vi "ChannelUI.vi"() -> ()   [LabVIEW 2014, in "Channel.lvclass"]
doc: "Template for creating new user-interface VIs for inherited classes."
uses:
  Channel.lvclass
  <vilib>/NI/AMC/Message Queue.ctl
  <vilib>/NI/AMC/Message.ctl
  <vilib>/NI/Tools/Keyed Array/KeyedArray.ctl
  xCE/xceTreeObj/xceTreeObj.lvclass
  channel_dataType.ctl
  _Shared/Symbols/enum_Symbols.ctl
  Channel.lvclass/Channel.ctl
  Channel_FXP/Channel_FXP.lvclass
  Channel_FXP/Channel_FXP.lvclass/Channel_FXP.ctl
  xCE/_shared/replaceNode.ctl
  xCE/xceDataNode/xceDataNode.lvclass
  <vilib>/NI/AMC/Read Termination Message.vi
  <vilib>/NI/AMC/Create Single Message.vi
  <vilib>/NI/AMC/Update Message Routing Info.vi
  <vilib>/NI/AMC/Globals.vi
  <vilib>/NI/AMC/Send Message.vi
  <vilib>/NI/AMC/AMC.lvlib
  xCE/xceNode/xceNode.lvclass
  <vilib>/NI/Tools/Keyed Array/Tools_KeyedArray.lvlib
panel:
  in  "View Mode":enum32{"Channel", "Parameter"}(tab)
  in  "Offset":dbl format="%#_12g"
  in  "Scale":dbl format="%#_12g"
  in  "Set Scale and Offset":bool
  in  "Description":string
  in  "Category":string="Default"
  in  "Name":string
  in  "Symbol":T1
  in  "Unit":string
  in  "Channel Specific":enum32{"Basic", "FXP"}(tab)
  in  "FXP Integer Length":i32
  in  "FXP - Word Length":i32
  in  "Parameter":T2
  in  "Data Type":T3
  in  "DataNode*":refnum<data-value>
  in  "AMC*":T4
  in  "Exit":bool
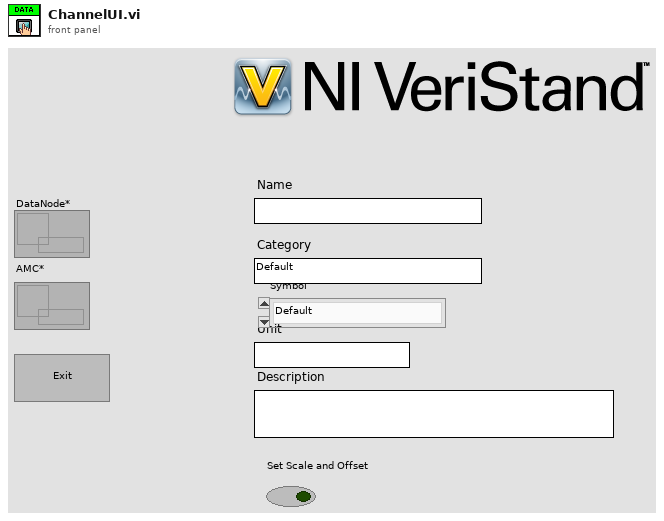
[diagram p1: front panel]
types:
  T1 = typedef "enum_Symbols.ctl" = enum16{"Default", "Analog Input", "Analog Output", "Digital Input", "Digital Output", "PWM Input", "PWM Output"}
  T2 = cluster{"Name":string, "Control Name":string, "Initial Value":dbl, "Scale":dbl, "Offset":dbl}
  T3 = typedef "Channel.lvclass/channel_dataType.ctl" = enum16{"Boolean", "U8", "I8", "U16", "I16", "U32", "I32", "U64", "I64", "FXPI32", "FXPU32", "FXPI64", "FXPU64", "PWM"}
  T4 = typedef "AMC.lvlib/Message Queue.ctl" = refnum<queue>
  T5 = typedef "replaceNode.ctl" = cluster{"ToReplaceNode*":refnum<data-value>, "Replace Class":string}
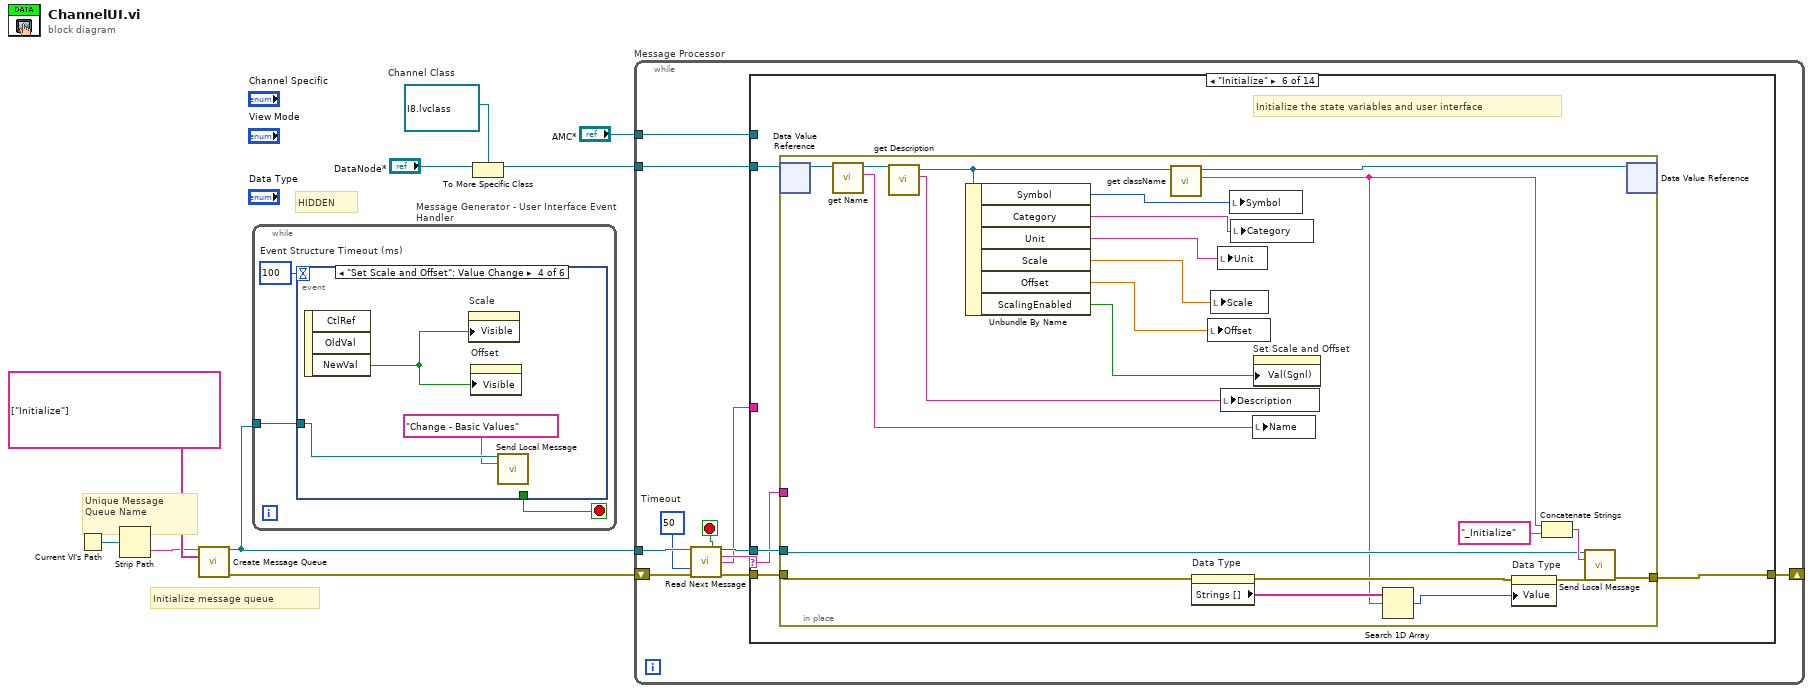
[diagram p0: block diagram]
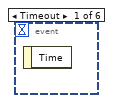
[diagram p2: hidden frame]
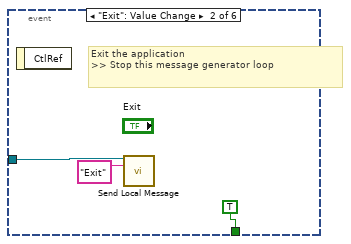
[diagram p3: hidden frame]
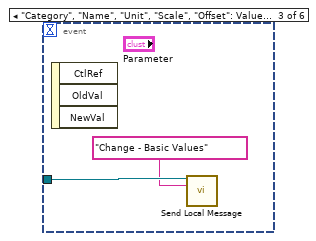
[diagram p4: hidden frame]
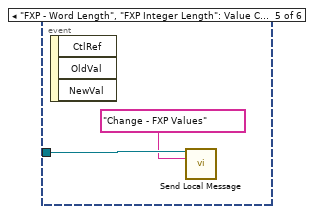
[diagram p5: hidden frame]
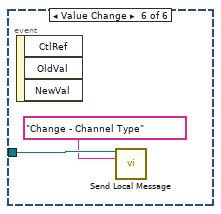
[diagram p6: hidden frame]
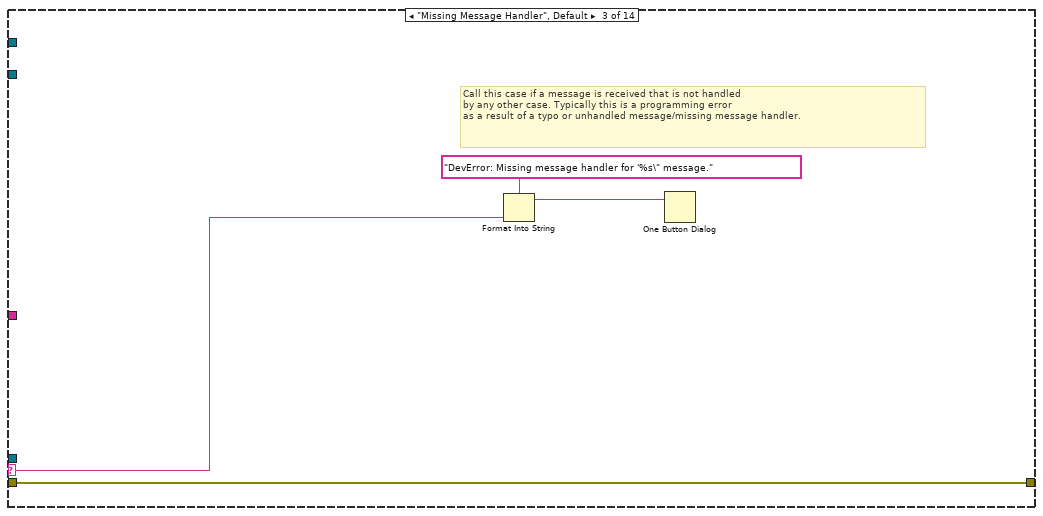
[diagram p9: hidden frame]
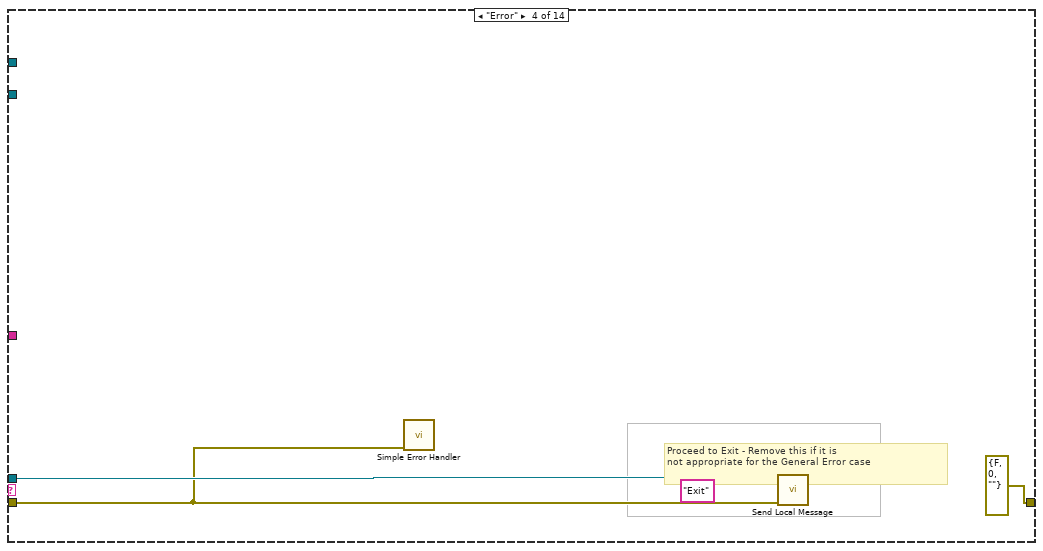
[diagram p10: hidden frame]
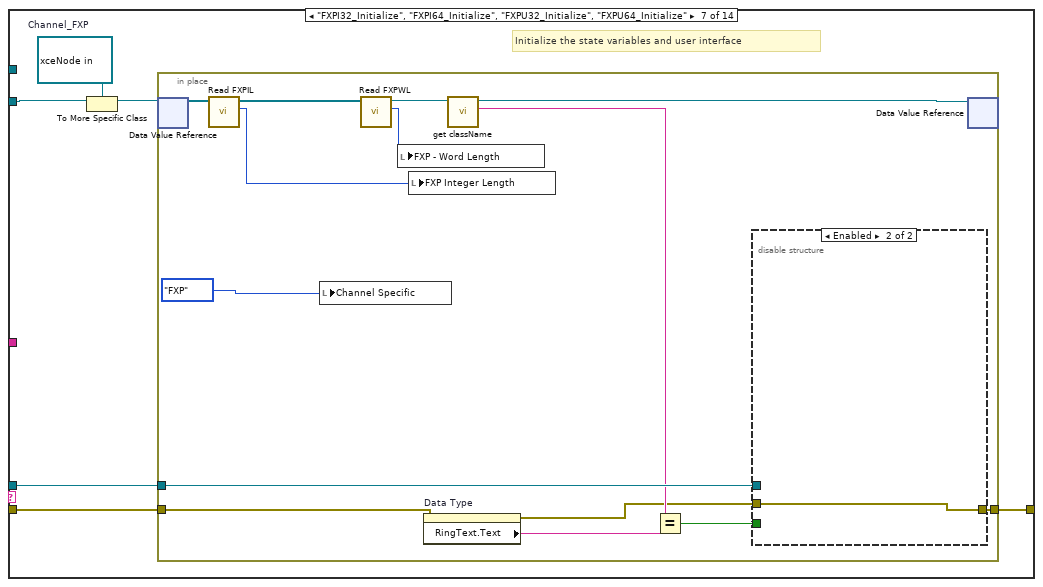
[diagram p12: hidden frame]
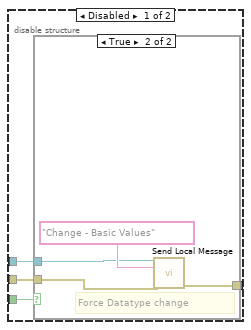
[diagram p13: hidden frame]
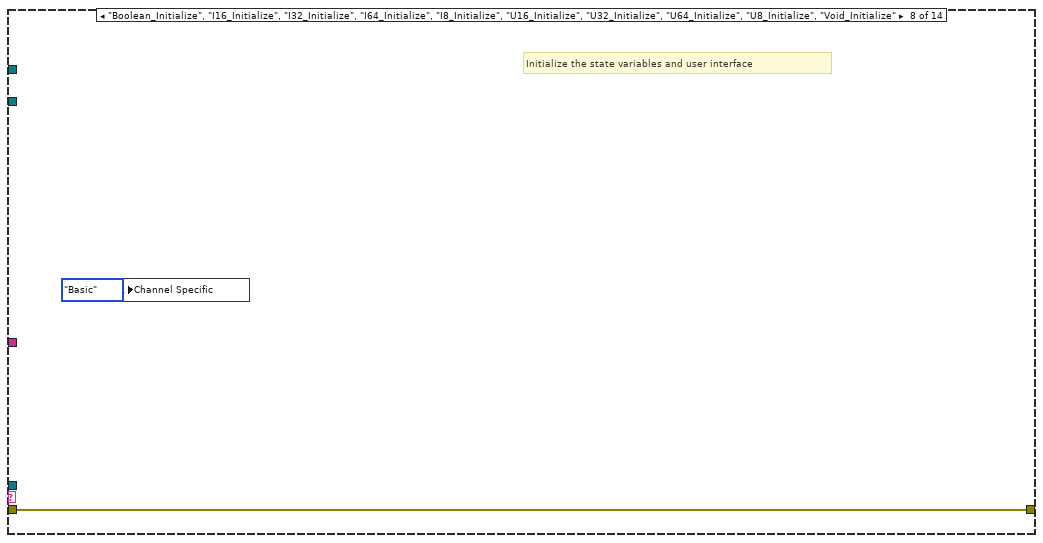
[diagram p15: hidden frame]
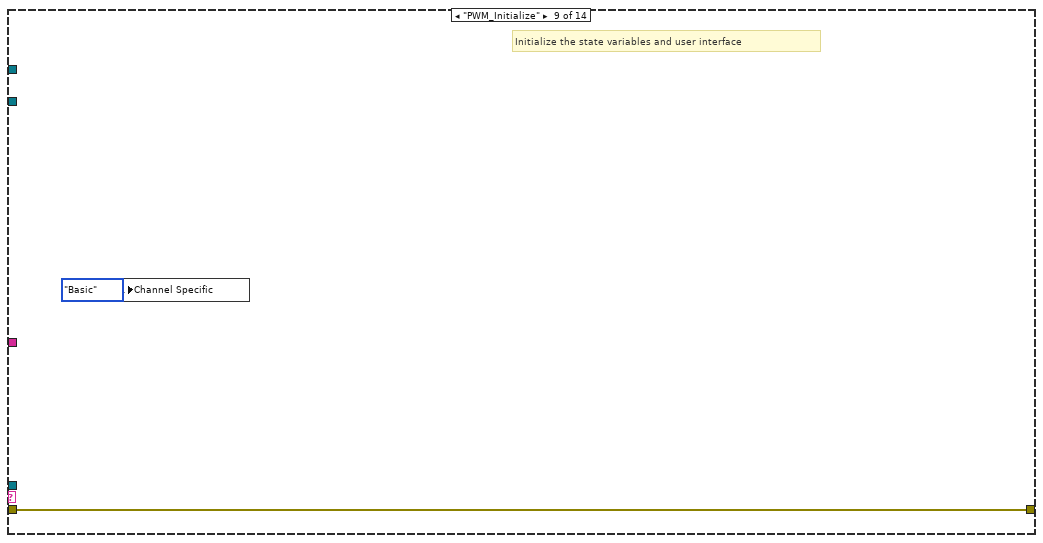
[diagram p16: hidden frame]
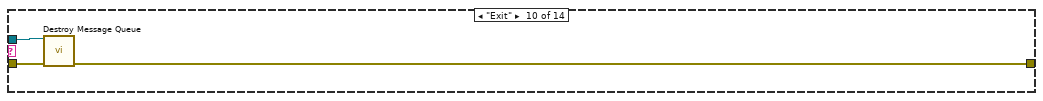
[diagram p17: hidden frame]
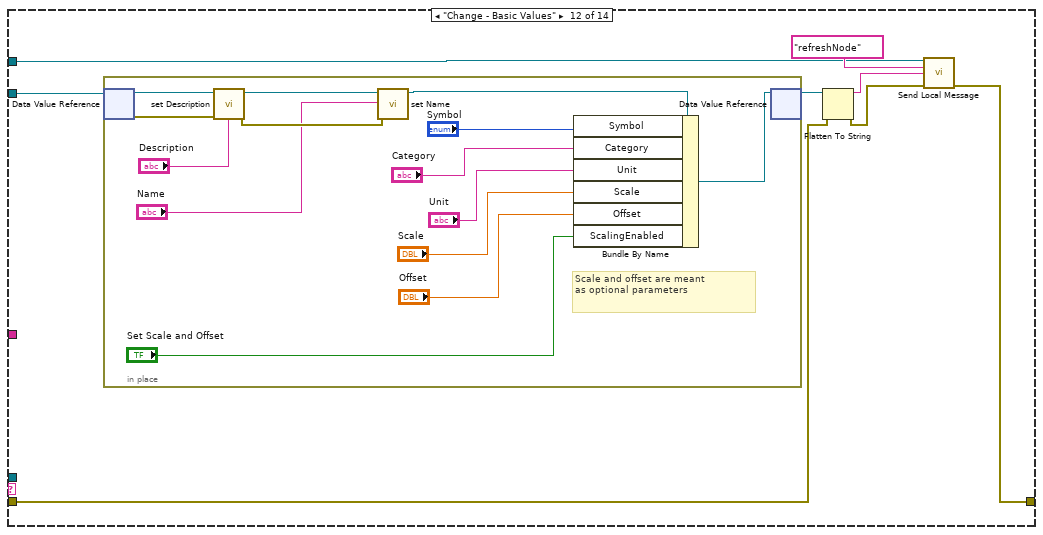
[diagram p19: hidden frame]
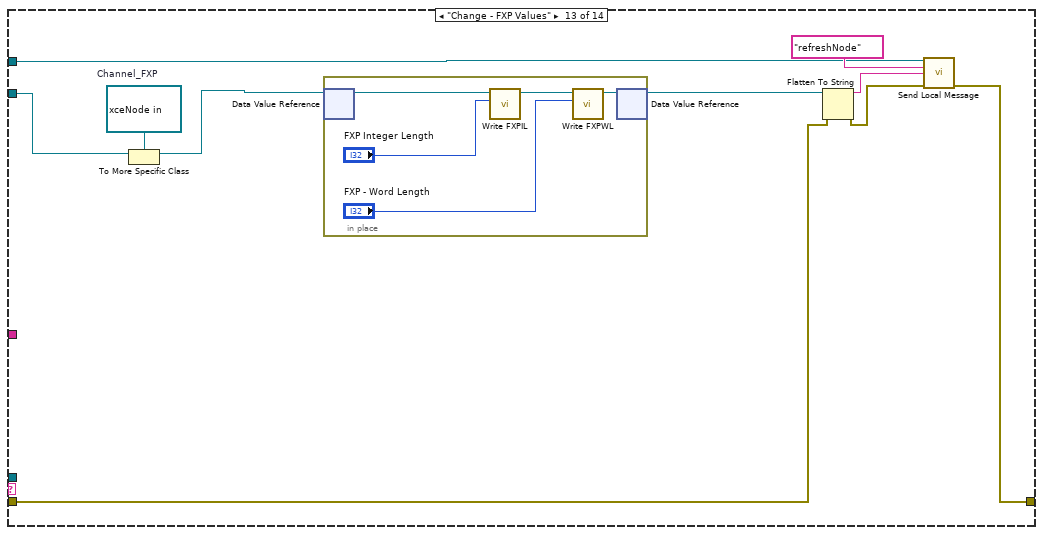
[diagram p20: hidden frame]
diagram:
  w1 = refnum<data-value> refnum  # Channel Class
  # "HIDDEN"
  # "Initialize message queue"
  # "Unique Message\nQueue Name"
  n1 = Current VI's Path() -> (path=w5:path)
  n2 = Strip Path(path=w5) -> (name=w8:string)  [unwired: 1 out]
  n3 = call <vilib>:"Create Message Queue.vi"("message queue name"=w8, "initial message names"=string[] ["Initialize"]) -> ("message queue out"=w7:T4, "error out"=w6:errorcluster)  [unwired: 12 in]
  n4 = while "Message Generator - User Interface Event Handler" {
    tunnel: w7 -> [w10]
    stop <- w11 stop-if-true
    w12 = 100  # Event Structure Timeout (ms)
    n5 = event shown="[3] \"Set Scale and Offset\": Value Change" {
      selector: _ -> [_ _ _ _ _ _]
      dyn-events: _ -> [_ _ _ _ _ _]
      timeout: w12 -> [_ _ _ _ _ _]
      tunnel: [_ TRUE ("Discard?") _ _ _ _] -> w11
      tunnel: w10 -> [_ w13 w17 w19 w22 w24]
      event Timeout {
        n6 = event-data() -> ()  [unwired: 2 out]
      }
      event "Exit": Value Change {
        # "Exit the application\n>> Stop this message generator loop"
        n7 = event-data() -> ()  [unwired: 2 out]
        n8 = call <vilib>:"Send Local Message.vi"("message queue in"=w13, "message name"="Exit") -> ()  [unwired: 11 in, 3 out]
      }
      event "Category", "Name", "Unit", "Scale", "Offset": Value Change {
        n9 = event-data() -> ()  [unwired: 4 out]
        n10 = call <vilib>:"Send Local Message.vi"("message queue in"=w17, "message name"="Change - Basic Values" ("Message Name")) -> ()  [unwired: 11 in, 3 out]
      }
      event "Set Scale and Offset": Value Change {
        n11 = event-data() -> ("NewVal"=w20:bool)  [unwired: 3 out]
        n12 = property on="Scale" class="DigNum (strict)"("Visible"=w20) -> ()  [unwired: 2 in, 2 out]
        n13 = property on="Offset" class="DigNum (strict)"("Visible"=w20) -> ()  [unwired: 2 in, 2 out]
        n14 = call <vilib>:"Send Local Message.vi"("message queue in"=w19, "message name"="Change - Basic Values" ("Message Name")) -> ()  [unwired: 11 in, 3 out]
      }
      event "FXP - Word Length", "FXP Integer Length": Value Change {
        n15 = event-data() -> ()  [unwired: 4 out]
        n16 = call <vilib>:"Send Local Message.vi"("message queue in"=w22, "message name"="Change - FXP Values" ("Message Name")) -> ()  [unwired: 11 in, 3 out]
      }
      event Value Change {
        n17 = event-data() -> ()  [unwired: 4 out]
        n18 = call <vilib>:"Send Local Message.vi"("message queue in"=w24, "message name"="Change - Channel Type" ("Message Name")) -> ()  [unwired: 11 in, 3 out]
      }
    }
  }
  n19 = To More Specific Class(target class=w1, reference="DataNode*") -> (specific class reference=w2:refnum<data-value>)  [unwired: 1 in, 1 out]
  n20 = while "Message Processor" {
    shift-left: w6 -> [w32]
    shift-right: [w25] -> _
    tunnel: w7 -> [w33]
    tunnel: "AMC*" -> [w26]
    tunnel: w2 -> [w27]
    stop <- w35 stop-if-true
    w30 = 50  # Timeout
    n21 = call <vilib>:"Read Next Message.vi"("message queue in"=w33, "timeout (1 ms)"=w30, "error in"=w32) -> ("exit process?"=w35:bool, "message queue out"=w34:T4, "message name"=w29:string, "message value"=w28:string, "error out"=w31:errorcluster)  [unwired: 5 in, 3 out]
    n22 = case shown="\"Initialize\"" w29 {
      selector: w29 -> [_ _ w41 _ _ w47 _ _ _ _ _ _ _ _]
      tunnel: w34 -> [_ _ _ w45 _ w49 w78 _ _ w109 _ _ _ _]
      tunnel: w31 -> [w36 w37 w38 w43 w46 w50 w79 w105 w107 w110 w111 w113 w138 w151]
      tunnel: w28 -> [_ _ _ _ _ _ _ _ _ _ _ _ _ _]
      tunnel: w27 -> [_ _ _ _ _ w51 w77 _ _ _ _ w119 w135 w157]
      tunnel: w26 -> [_ _ _ _ _ _ _ _ _ _ _ w115 w140 w155]
      tunnel: [w36 w37 w38 errorcluster {"status"=FALSE, "code"=0, "source"=""} ("error out") w46 w48 w74 w105 w107 w108 w111 w112 w137 w152] -> w25
      frame "---------- Framework Operations ----------" {
        # "Dummy case to add a seperator in the Case Structure menu"
      }
      frame "", "Idle" {
      }
      frame "Missing Message Handler", Default {
        # "Call this case if a message is received that is not handled \nby any other case. Typically this is a programming error\nas a result of a typo or unhandled message/missing message handler."
        n23 = Format Into String(format string="DevError: Missing message handler for '%s\" message." ("message"), w41) -> (resulting string=w39:string)  [unwired: 2 in, 1 out]
        n24 = One Button Dialog(message=w39) -> ()  [unwired: 2 out]
      }
      frame "Error" {
        # "Proceed to Exit - Remove this if it is\nnot appropriate for the General Error case"
        n25 = call <vilib>:"Simple Error Handler.vi"("error in (no error)"=w43) -> ()  [unwired: 1 in, 8 out]
        n26 = call <vilib>:"Send Local Message.vi"("message queue in"=w45, "message name"="Exit", "error in"=w43) -> ()  [unwired: 10 in, 3 out]
      }
      frame "---------- Generic Operations ----------" {
        # "Dummy case to add a seperator in the Case Structure menu"
      }
      frame "Initialize" {
        # "Initialize the state variables and user interface"
        n27 = in-place {
          in-place-border: w50 -> [w60]
          in-place-border: w49 -> [w62]
          in-place-border: [w61] -> w48
          in-place-border: w47 -> [_]
          n28 = in-place-dvr #1(w51) -> (w68:refnum<class "Channel.lvclass">)  [unwired: 1 out]
          n29 = call "get Name.vi"("xceDataNode in"=w68) -> ("Name"=w72:string, "xceDataNode out"=w73:refnum<class "Channel.lvclass">)  [unwired: 8 in, 1 out]
          n30 = call "get Description.vi"("xceDataNode in"=w73) -> ("Description"=w71:string, "xceDataNode out"=w67:refnum<class "Channel.lvclass">)  [unwired: 8 in, 1 out]
          n31 = Unbundle By Name(w67) -> ("Symbol"=w70:T1, "Category"=w69:string, "Unit"=w65:string, "Scale"=w53:dbl, "Offset"=w54:dbl, "ScalingEnabled"=w52:bool)
          n32 = call "get className.vi"("xceNode in"=w67) -> ("Class name"=w55:string, "xceNode out"=w66:refnum<class "Channel.lvclass">)  [unwired: 8 in, 1 out]
          n33 = property on="Data Type" class="Enum (strict)"(error in=w60) -> (error out=w58:errorcluster, "Strings []"=w59:string[])  [unwired: 1 in, 1 out]
          n34 = local write "Offset"(w54) -> ()
          n35 = local write "Scale"(w53) -> ()
          n36 = local write "Unit"(w65) -> ()
          n37 = local write "Description"(w71) -> ()
          n38 = local write "Symbol"(w70) -> ()
          n39 = local write "Category"(w69) -> ()
          n40 = local write "Name"(w72) -> ()
          n41 = property on="Set Scale and Offset" class="Bool (strict)"("Val(Sgnl)"=w52) -> ()  [unwired: 2 in, 2 out]
          n42 = Search 1D Array(1D array=w59, element=w55) -> (index of element=w57:i32)  [unwired: 1 in]
          n43 = property on="Data Type" class="Enum (strict)"(error in=w58, "Value"=w57) -> (error out=w56:errorcluster)  [unwired: 1 in, 1 out]
          n44 = Concatenate Strings(w55, "_Initialize" ("string")) -> (w63:string)
          n45 = call <vilib>:"Send Local Message.vi"("message queue in"=w62, "message name"=w63, "error in"=w56) -> ("error out"=w61:errorcluster)  [unwired: 10 in, 2 out]
          n46 = in-place-dvr #1(w66) -> ()  [unwired: 2 out]
        }
      }
      frame "FXPI32_Initialize", "FXPI64_Initialize", "FXPU32_Initialize", "FXPU64_Initialize" {
        w76 = refnum<data-value> refnum  # Channel_FXP
        # "Initialize the state variables and user interface"
        n47 = To More Specific Class(target class=w76, reference=w77) -> (specific class reference=w75:refnum<data-value>)  [unwired: 1 in, 1 out]
        n48 = in-place {
          in-place-border: w79 -> [w90]
          in-place-border: w78 -> [w89]
          in-place-border: [w84] -> w74
          n49 = in-place-dvr #2(w75) -> (w93:refnum<class "Channel_FXP.lvclass">)  [unwired: 1 out]
          n50 = call "Read FXPIL.vi"("Channel_FXP in"=w93) -> ("FXPIL"=w81:i32, "Channel_FXP out"=w92:refnum<class "Channel_FXP.lvclass">)  [unwired: 8 in, 1 out]
          n51 = local write "Channel Specific"(enum32{"Basic", "FXP"}."FXP" ("Tab Control")) -> ()
          n52 = call "Read FXPWL.vi"("Channel_FXP in"=w92) -> ("FXPWL"=w80:i32, "Channel_FXP out"=w91:refnum<class "Channel_FXP.lvclass">)  [unwired: 8 in, 1 out]
          n53 = local write "FXP - Word Length"(w80) -> ()
          n54 = local write "FXP Integer Length"(w81) -> ()
          n55 = property on="Data Type" class="Enum (strict)"(error in=w90) -> (error out=w85:errorcluster, "RingText.Text"=w88:string)  [unwired: 1 in, 1 out]
          n56 = call "get className.vi"("xceNode in"=w91) -> ("Class name"=w87:string, "xceNode out"=w83:refnum<class "Channel_FXP.lvclass">)  [unwired: 8 in, 1 out]
          n57 = Equal?(x=w87, y=w88) -> (x = y?=w86:bool)
          n58 = disable-structure shown="Enabled" {
            disable-tunnel: w89 -> [w97 _]
            disable-tunnel: w86 -> [w96 _]
            disable-tunnel: w85 -> [w95 w103]
            disable-tunnel: [w94 w103] -> w84
            frame Disabled {
              n59 = case shown="True" w96 {
                tunnel: [w98 w101] -> w94
                tunnel: w97 -> [_ w100]
                tunnel: w95 -> [w98 w99]
                frame False {
                }
                frame True {
                  # "Force Datatype change"
                  n60 = call <vilib>:"Send Local Message.vi"("message queue in"=w100, "message name"="Change - Basic Values" ("Message Name"), "error in"=w99) -> ("error out"=w101:errorcluster)  [unwired: 10 in, 2 out]
                }
              }
            }
            frame Enabled {
            }
          }
          n61 = in-place-dvr #2(w83) -> ()  [unwired: 2 out]
        }
      }
      frame "Boolean_Initialize", "I16_Initialize", "I32_Initialize", "I64_Initialize", "I8_Initialize", "U16_Initialize", "U32_Initialize", "U64_Initialize", "U8_Initialize", "Void_Initialize" {
        # "Initialize the state variables and user interface"
        n62 = local write "Channel Specific"(enum32{"Basic", "FXP", "PWM"}."Basic" ("Channel Specific")) -> ()
      }
      frame "PWM_Initialize" {
        # "Initialize the state variables and user interface"
        n63 = local write "Channel Specific"(enum32{"Basic", "FXP", "PWM"}."Basic" ("Channel Specific")) -> ()
      }
      frame "Exit" {
        n64 = call <vilib>:"Destroy Message Queue.vi"("message queue in"=w109, "error in"=w110) -> ("error out"=w108:errorcluster)  [unwired: 11 in, 2 out]
      }
      frame "---------- Application Operations ----------" {
        # "Dummy case to add a seperator in the Case Structure menu"
      }
      frame "Change - Basic Values" {
        n65 = in-place {
          # "Scale and offset are meant\nas optional parameters"
          n66 = in-place-dvr #3(w119) -> (w126:refnum<class "Channel.lvclass">, w125:errorcluster)
          n67 = call "set Description.vi"("error in (no error)"=w125, "Description"="Description", "xceDataNode in"=w126) -> ("error out"=w129:errorcluster, "xceDataNode out"=w130:refnum<class "Channel.lvclass">)  [unwired: 7 in]
          n68 = call "set Name.vi"("error in (no error)"=w129, "Name"="Name", "xceDataNode in"=w130) -> ("xceDataNode out"=w128:refnum<class "Channel.lvclass">)  [unwired: 7 in, 1 out]
          n69 = Bundle By Name(cluster=w128, "Symbol"="Symbol", "Category"="Category", "Unit"="Unit", "Scale"="Scale", "Offset"="Offset", "ScalingEnabled"="Set Scale and Offset") -> (w133:refnum<class "Channel.lvclass">)
          n70 = in-place-dvr #3(w133) -> (w114:refnum<data-value>)  [unwired: 1 out]
        }
        n71 = Flatten To String(anything=w114, error in (no error)=w113) -> (data string=w118:string, error out=w116:errorcluster)  [unwired: 2 in, 1 out]
        n72 = call <vilib>:"Send Local Message.vi"("message queue in"=w115, "message name"="refreshNode" ("Message Name"), "message value"=w118, "error in"=w116) -> ("error out"=w112:errorcluster)  [unwired: 9 in, 2 out]
      }
      frame "Change - FXP Values" {
        w136 = refnum<data-value> refnum  # Channel_FXP
        n73 = To More Specific Class(target class=w136, reference=w135) -> (specific class reference=w134:refnum<data-value>)  [unwired: 1 in, 1 out]
        n74 = in-place {
          n75 = in-place-dvr #4(w134) -> (w148:refnum<class "Channel_FXP.lvclass">)  [unwired: 1 out]
          n76 = call "Write FXPIL.vi"("FXPIL"="FXP Integer Length", "Channel_FXP in"=w148) -> ("Channel_FXP out"=w147:refnum<class "Channel_FXP.lvclass">)  [unwired: 8 in, 1 out]
          n77 = call "Write FXPWL.vi"("FXPWL"="FXP - Word Length", "Channel_FXP in"=w147) -> ("Channel_FXP out"=w146:refnum<class "Channel_FXP.lvclass">)  [unwired: 8 in, 1 out]
          n78 = in-place-dvr #4(w146) -> (w139:refnum<data-value>)  [unwired: 1 out]
        }
        n79 = Flatten To String(anything=w139, error in (no error)=w138) -> (data string=w143:string, error out=w141:errorcluster)  [unwired: 2 in, 1 out]
        n80 = call <vilib>:"Send Local Message.vi"("message queue in"=w140, "message name"="refreshNode" ("Message Name"), "message value"=w143, "error in"=w141) -> ("error out"=w137:errorcluster)  [unwired: 9 in, 2 out]
      }
      frame "Change - Channel Type" {
        w158 = T5 {"ToReplaceNode*"=refnum, "Replace Class"=""}  # replaceNode
        n81 = property on="Data Type" class="Enum (strict)"(error in=w151) -> (error out=w150:errorcluster, "RingText.Text"=w149:string)  [unwired: 1 in, 1 out]
        n82 = Bundle By Name(cluster=w158, "ToReplaceNode*"=w157, "Replace Class"=w149) -> (w156:T5)
        n83 = Flatten To String(anything=w156) -> (data string=w153:string)  [unwired: 3 in, 2 out]
        n84 = call <vilib>:"Send Local Message.vi"("message queue in"=w155, "message name"="replaceNode" ("Message Name"), "message value"=w153, "error in"=w150) -> ("error out"=w152:errorcluster)  [unwired: 9 in, 2 out]
      }
    }
  }
